vi "escribeGaugeFrec.vi"(1 "Fin":sgl) -> (0 "Frec out":cluster{"Max":sgl, "Vin":sgl, "Min":sgl})   [LabVIEW 2018]
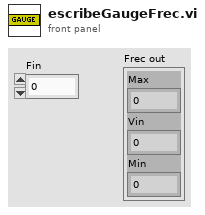
[diagram p1: front panel]
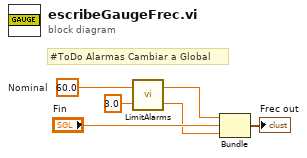
[diagram p0: block diagram]
diagram:
  w2 = sgl 60.0  # Nominal
  # "#ToDo Alarmas Cambiar a Global"
  n1 = call "LimitAlarms.vi"("Value"=sgl 3.0, "Parameter"=w2) -> ("Min"=w5:sgl, "Max"=w4:sgl)
  n2 = Bundle("Max"=w4, "Fin"="Fin", "Min"=w5) -> (→"Frec out":cluster{"Max":sgl, "Fin":sgl, "Min":sgl})  [unwired: 1 in]
